vi "LEBITVacuum.UpdateQuality.vi"(0 "i ref in":refnum<vi>, 1 "data":i16, 2 "i attribute":T4={"setValuePLC"=[], "nickNames"=[], "setValuePLCServiceID"=[], "monValuePLC"=[], "SetValueServiceID"=[], "MonValueServiceID"=[], "SetValue"=[], "AllPLCValues"=[], "CondSpecial2DArray"=[], "CondSpecialIndex"=[], "ReasonForLocking"="", "ReasonForLockingID"=0, "enableValuePLC"=[], "OverwriteCloseSafetyPLC"=[], "OverwriteOpenSafetyPLC"=[], "OverwriteCloseSafetyPLCServiceID"=[], "OverwriteOpenSafetyPLCServiceID"=[], "MKS Address Array"=[], "MKS MeasurementServiceID"=[], "MKS Measurement"=[], "CRYO Measurement"=[], "CRYO MeasurementServiceID"=[], "Special"=[], "Start Date"="", "MKS VISA resource"="COM13", "CRYO VISA resource"="COM13"}, 3 "index":i32, 5 "error in":errorcluster, 6 "quality":i32, 9 "no link":bool) -> (14 "i ref out":refnum<vi>, 16 "i attribute out":T4={"setValuePLC"=[], "nickNames"=[], "setValuePLCServiceID"=[], "monValuePLC"=[], "SetValueServiceID"=[], "MonValueServiceID"=[], "SetValue"=[], "AllPLCValues"=[], "CondSpecial2DArray"=[], "CondSpecialIndex"=[], "ReasonForLocking"="", "ReasonForLockingID"=0, "enableValuePLC"=[], "OverwriteCloseSafetyPLC"=[], "OverwriteOpenSafetyPLC"=[], "OverwriteCloseSafetyPLCServiceID"=[], "OverwriteOpenSafetyPLCServiceID"=[], "MKS Address Array"=[], "MKS MeasurementServiceID"=[], "MKS Measurement"=[], "CRYO Measurement"=[], "CRYO MeasurementServiceID"=[], "Special"=[], "Start Date"="", "MKS VISA resource"="COM13", "CRYO VISA resource"="COM13"}, 19 "error out":errorcluster)   [LabVIEW 2014, in "LEBITVacuum.lvlib"]
uses:
  LEBITVacuum.lvlib
  LEBITVacuum.i attribute.ctl
  CSCore/CSSystem/CoreDefs/CoreDefs.call_type.ctl
  CSCore/BaseProcess/BaseProcess.descriptor string definition.ctl
  CSCore/CSSystem/CoreDefs/CoreDefs.rawDataType.ctl
  CSlibraries/UtilityLib/UtilityLib.valueStatus.ctl
  CSCore/CSSystem/CoreLib/CoreLib.string 2 byte array.vi
  CSCore/CSSystem/CoreLib/CoreLib.byte array 2 short.vi
  CSlibraries-extern/DimLVEvent/LVDimInterface/LVDimInterface.lvlib
  CSCore/CSSystem/CoreLib/CoreLib.lvlib
  CSlibraries/UtilityLib/UtilityLib.lvlib
  CSCore/BaseProcess/BaseProcess.lvlib
panel:
  in  "call cluster in":T1={"Object"="", "Selector"="", "CallType"=enum."synchronous", "Async Object"="", "Async Selector"="", "Data Descriptor"="", "Data"=[], "Error #"=0, "Expire"=0}
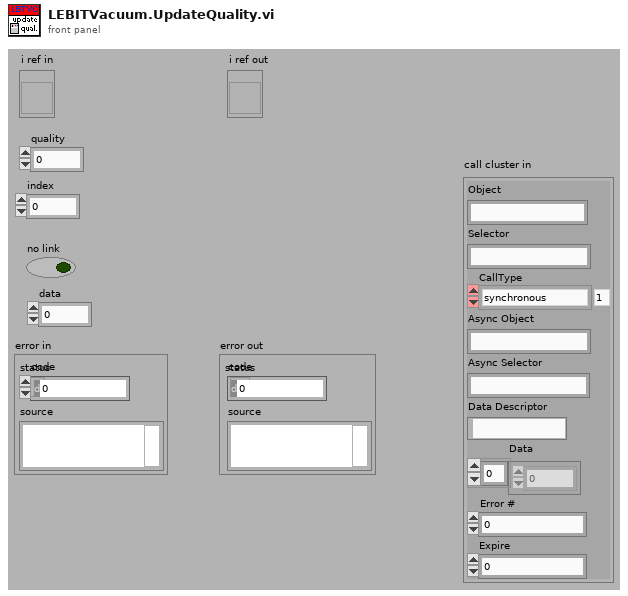
[diagram p1: front panel]
types:
  T1 = typedef "CoreDefs.call_type.ctl" = cluster{"Object":string, "Selector":string, "CallType":enum16{"simple", "synchronous", "asynchronous"}, "Async Object":string, "Async Selector":string, "Data Descriptor":T2, "Data":T3, "Error #":i32, "Expire":u32}
  T2 = typedef "BaseProcess.lvlib/BaseProcess.descriptor string definition.ctl" = string
  T3 = typedef "CoreDefs.rawDataType.ctl" = i8[]
  T4 = typedef "LEBITVacuum.lvlib/LEBITVacuum.i attribute.ctl" = cluster{"setValuePLC":string[], "nickNames":string[], "setValuePLCServiceID":i32[], "monValuePLC":string[], "SetValueServiceID":i32[], "MonValueServiceID":i32[], "SetValue":i16[], "AllPLCValues":string[], "CondSpecial2DArray":string[][], "CondSpecialIndex":i32[], "ReasonForLocking":string, "ReasonForLockingID":i32, "enableValuePLC":string[], "OverwriteCloseSafetyPLC":string[], "OverwriteOpenSafetyPLC":string[], "OverwriteCloseSafetyPLCServiceID":i32[], "OverwriteOpenSafetyPLCServiceID":i32[], "MKS Address Array":i32[][], "MKS MeasurementServiceID":i32[], "MKS Measurement":string[], "CRYO Measurement":string[][], "CRYO MeasurementServiceID":i32[], "Special":string[], "Start Date":string, "MKS VISA resource":refnum<visa-resource-name>, "CRYO VISA resource":refnum<visa-resource-name>}
  T5 = typedef "UtilityLib.lvlib/UtilityLib.valueStatus.ctl" = enum16{"no info available", "stand by/off", "on", "warning", "alarm/malfunction", "not implemented", "user action required", "important information", "system default", "control default", "indicator default", "button default"}
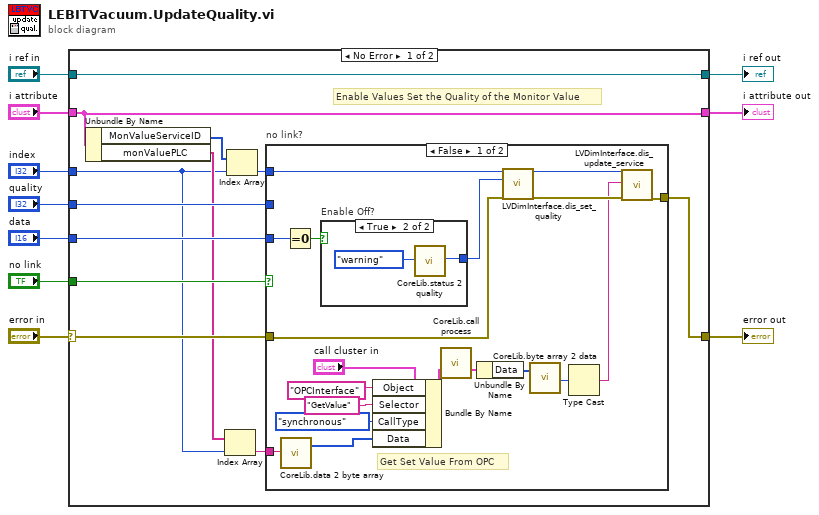
[diagram p0: block diagram]
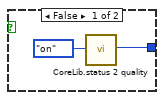
[diagram p2: hidden frame]
diagram:
  n1 = case shown="No Error" "error in" {
    selector: "error in" -> [w17 w49]
    tunnel: "quality" -> [w22 _]
    tunnel: "no link" -> [w21 _]
    tunnel: [w16 w49] -> w8
    tunnel: "data" -> [w20 _]
    tunnel: "i attribute" -> [w15 w47]
    tunnel: "i ref in" -> [w14 w48]
    tunnel: [w14 w48] -> w4
    tunnel: "index" -> [w12 _]
    tunnel: [w15 w47] -> w2
    frame No Error {
      # "Enable Values Set the Quality of the Monitor Value"
      n2 = Unbundle By Name(w15) -> ("MonValueServiceID"=w19:i32[], "monValuePLC"=w13:string[])
      n3 = Index Array(array=w13, index=w12) -> (element=w11:string)
      n4 = Index Array(array=w19, index=w12) -> (element=w18:i32)
      n5 = case "no link?" shown="False" w21 {
        tunnel: w20 -> [w40 _]
        tunnel: w22 -> [_ _]
        tunnel: w18 -> [w38 _]
        tunnel: w17 -> [w41 w46]
        tunnel: [w35 w46] -> w16
        tunnel: w11 -> [w25 _]
        frame False {
          # "Get Set Value From OPC"
          n6 = call-poly "CoreLib.data 2 byte array.vi"("string"=w25) -> ("byteArray out"=w30:T3)  [unwired: 18 in]
          n7 = Equal To 0?(x=w40) -> (x = 0?=w39:bool)
          n8 = case "Enable Off?" shown="True" w39 {
            tunnel: [w42 w44] -> w34
            frame False {
              n9 = call "CoreLib.status 2 quality.vi"("valueStatus"=UtilityLib.valueStatus."on") -> ("quality"=w42:i32)  [unwired: 18 in]
            }
            frame True {
              n10 = call "CoreLib.status 2 quality.vi"("valueStatus"=UtilityLib.valueStatus."warning") -> ("quality"=w44:i32)  [unwired: 18 in]
            }
          }
          n11 = Bundle By Name(cluster="call cluster in", "Object"="OPCInterface", "Selector"="GetValue" ("string"), "CallType"=enum16{"simple", "synchronous", "asynchronous"}."synchronous", "Data"=w30) -> (w33:T1)
          n12 = call "CoreLib.call process.vi"("call cluster in"=w33) -> ("call cluster out"=w27:T1)  [unwired: 13 in, 1 out]
          n13 = Unbundle By Name(w27) -> ("Data"=w26:T3)
          n14 = call "LVDimInterface.dis_set_quality.vi"("my_serviceID"=w38, "quality"=w34, "error in (no error)"=w41) -> ("my_serviceID (out)"=w37:i32, "error out"=w36:errorcluster)  [unwired: 15 in]
          n15 = call-poly "CoreLib.byte array 2 data.vi"("byteArray"=w26) -> ("i16"=w24:i16)  [unwired: 16 in, 2 out]
          n16 = Type Cast(x=w24) -> (*(type *) &x=w23:string)  [unwired: 1 in]
          n17 = call "LVDimInterface.dis_update_service.vi"("my_serviceID"=w37, "data"=w23, "error in (no error)"=w36) -> ("error out"=w35:errorcluster)  [unwired: 14 in, 2 out]
        }
        frame True {
        }
      }
    }
    frame Error {
    }
  }
  "error out" <- w8
  "i ref out" <- w4
  "i attribute out" <- w2
